vi "Logic_Open_Connection.vi"(4 "error in (no error)":errorcluster, 5 "Port [10430]":i32=10430, 6 "IP Address [127.0.0.1]":string="127.0.0.1", 7 "Python Session In":refnum<k35>) -> (0 "error out":errorcluster, 3 "Session Ref Out":T1)   [LabVIEW 2023]
doc: "Open connection to the Saleae Logic2 software."
panel:
  out "Expected Module Path":path
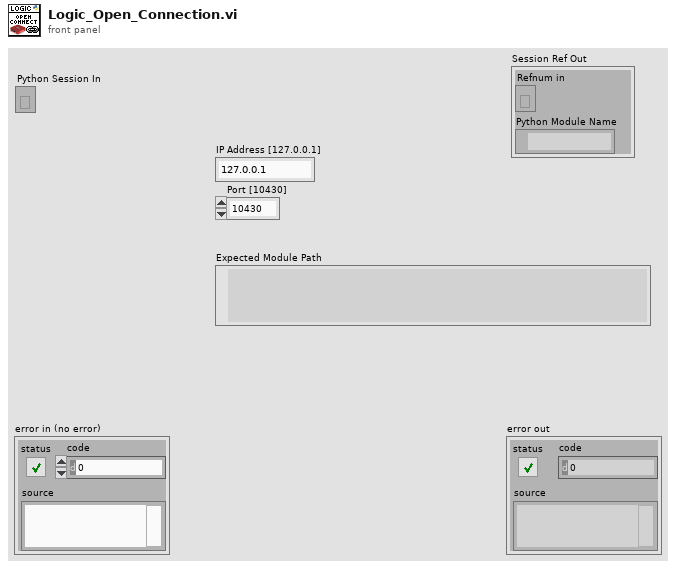
[diagram p1: front panel]
types:
  T1 = cluster{"Refnum in":refnum<k35>, "Python Module Name":path}
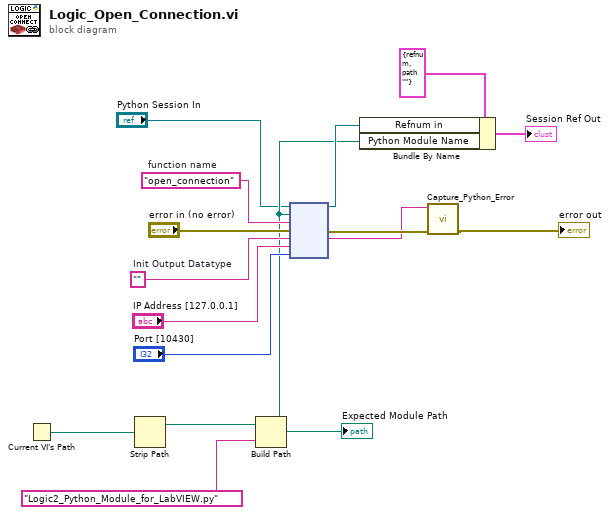
[diagram p0: block diagram]
diagram:
  w15 = "open_connection"  # function name
  w14 = ""  # Init Output Datatype
  n1 = Current VI's Path() -> (path=w8:path)
  n2 = Strip Path(path=w8) -> (stripped path=w4:path)  [unwired: 1 out]
  n3 = Build Path(base path=w4, name or relative path="Logic2_Python_Module_for_LabVIEW.py") -> (appended path=w7:path)
  "Expected Module Path" <- w7
  n4 = node("Python Session In", w7, w15, "error in (no error)", w14, "IP Address [127.0.0.1]", "Port [10430]") -> (w13:refnum<k35>, w2:errorcluster, w1:string)  [unwired: 2 in, 2 out]
  n5 = Bundle By Name(cluster=T1 {"Refnum in"=refnum, "Python Module Name"=path ""} ("output cluster"), "Refnum in"=w13, "Python Module Name"=w7) -> (→"Session Ref Out":T1)
  n6 = call "Capture_Python_Error.vi"("error in (no error)"=w2, "Error Message (start with ERROR)"=w1) -> ("error out"=→"error out":errorcluster)  [unwired: 9 in]
